vi "Multiply Float SCTL 40 MHz Latency 1.vi"(1 "y":sgl, 2 "x":sgl) -> (0 "x[k-1]*y[k-1]":sgl)   [LabVIEW 2017]
uses:
  <vilib>/rvi/IPIntegrationNode/IPINode_Typedef/niFpgaIPINodeSupportedFamilies.ctl
  <vilib>/rvi/IPIntegrationNode/IPINode_Utilities/niFpgaIPINodeSimCore.vi
  <vilib>/rvi/XilinxIP/XIPIN_XNode/niFpgaXIPIN.xnode
  Multiply SCTL L1/Multiply_SCTL_L1_C3ADE5BE76064AA39E7EE6565DE88692.dll
  <vilib>/rvi/IPIntegrationNode/IPINode_Xnode/niFpgaIPINode.xnode
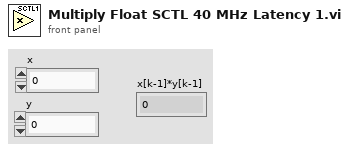
[diagram p1: front panel]
types:
  T1 = typedef "niFpgaIPINodeSupportedFamilies.ctl" = cluster{"unlimited?":bool, "supported targets":string[]}
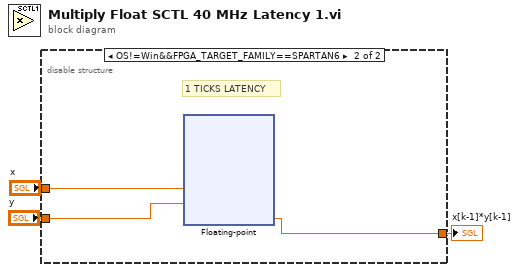
[diagram p0: block diagram]
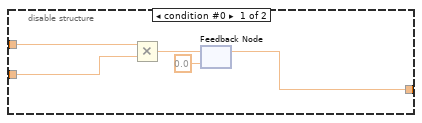
[diagram p2: hidden frame]
diagram:
  n1 = disable-structure shown="OS!=Win&&FPGA_TARGET_FAMILY==SPARTAN6" {
    disable-tunnel: "x" -> [w8 w11]
    disable-tunnel: "y" -> [w7 w10]
    disable-tunnel: [w5 w9] -> w1
    frame condition #0 {
      n2 = Multiply(x=w8, y=w7) -> (x*y=w6:sgl)
      n3 = feedback-in #1(w6) -> ()
      n4 = feedback #1(sgl 0.0) -> (w5:sgl)
    }
    frame condition #1 (active) {
      # "1 TICKS LATENCY"
      n5 = xnode ("Floating-point")("a"=w11, "b"=w10) -> ("result"=w9:sgl)  [unwired: 2 in]
    }
  }
  "x[k-1]*y[k-1]" <- w1
